vi "Set Window Width.vi"(0 "VI in":refnum<vi>, 7 "Width":i16, 11 "error in (no error)":errorcluster) -> (4 "VI out":refnum<vi>, 15 "error out":errorcluster)   [LabVIEW 2020]
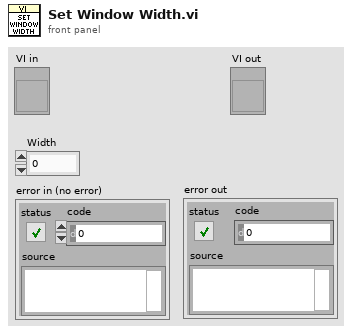
[diagram p1: front panel]
types:
  T1 = typedef "LVRectTypeDef.ctl" = cluster{"Left":i16, "Top":i16, "Right":i16, "Bottom":i16}
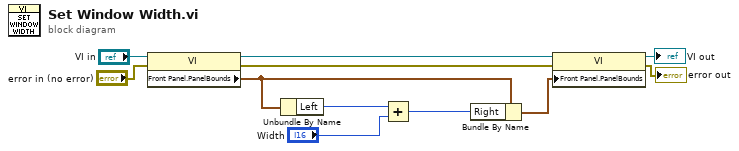
[diagram p0: block diagram]
diagram:
  n1 = property class="VI"(reference="VI in", error in="error in (no error)") -> (reference out=w6:refnum<vi>, error out=w8:errorcluster, "Front Panel.PanelBounds"=w11:T1)
  n2 = Unbundle By Name(w11) -> ("Left"=w3:i16)
  n3 = Add(x=w3, y="Width") -> (x+y=w9:i16)
  n4 = Bundle By Name(cluster=w11, "Right"=w9) -> (w10:T1)
  n5 = property class="VI"(reference=w6, error in=w8, "Front Panel.PanelBounds"=w10) -> (reference out=→"VI out":refnum<vi>, error out=→"error out":errorcluster)
